vi "RecibirDatosFireBase.vi"() -> ()   [LabVIEW 2025]
uses:
  <vilib>/httpClient/LabVIEWHTTPClient.lvlib
panel:
  out "rele":bool
  out "hora":string
  out "fecha":string
  out "accionamiento":dbl
  out "body":string
  out "headers":string
  out "error out":errorcluster
  in  "stop":bool
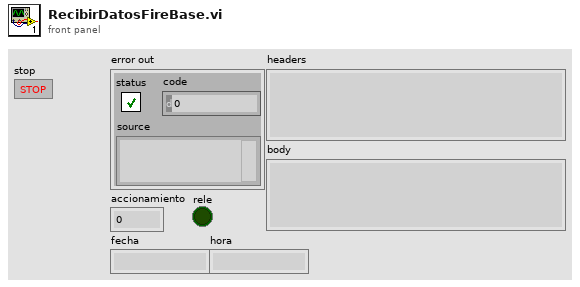
[diagram p1: front panel]
types:
  T1 = cluster{"accionamiento":dbl, "fecha":string, "hora":string, "rele":bool}
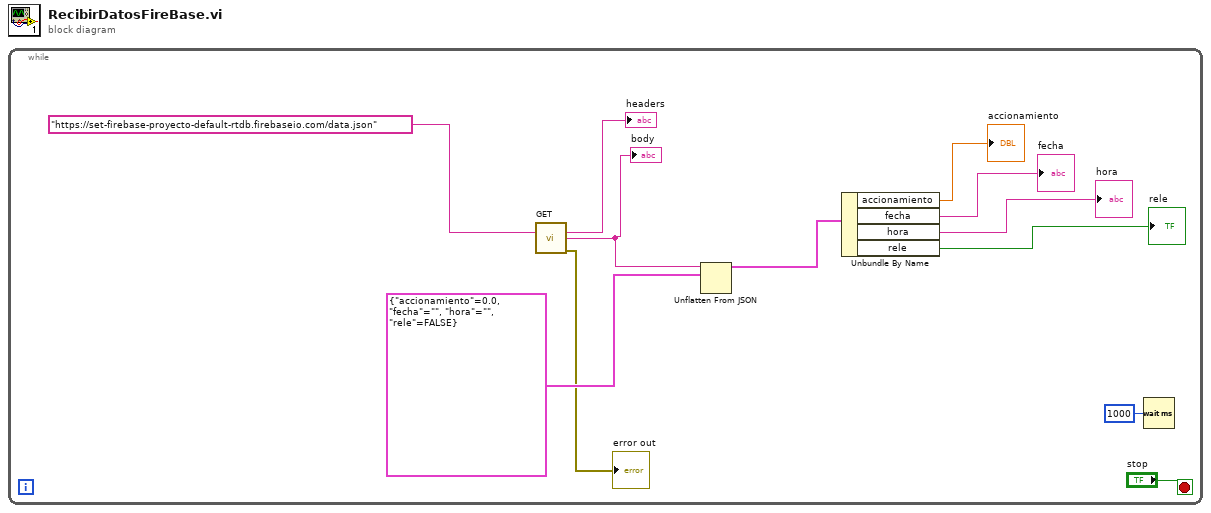
[diagram p0: block diagram]
diagram:
  n1 = while {
    stop <- "stop" stop-if-true
    n2 = call <vilib>:"GET.vi"("url"="https://set-firebase-proyecto-default-rtdb.firebaseio.com/data.json") -> ("headers"=→"headers":string, "body"=w6:string, "error out"=→"error out":errorcluster)  [unwired: 11 in, 1 out]
    "body" <- w6
    n3 = Unflatten From JSON(JSON string=w6, type and defaults=T1 {"accionamiento"=0.0, "fecha"="", "hora"="", "rele"=FALSE}) -> (value=w5:T1)  [unwired: 5 in, 1 out]
    n4 = Unbundle By Name(w5) -> ("accionamiento"=→"accionamiento":dbl, "fecha"=→"fecha":string, "hora"=→"hora":string, "rele"=→"rele":bool)
    n5 = Wait (ms)(milliseconds to wait=u32 1000) -> ()  [unwired: 1 out]
  }
